vi "Fit_and_Size.vi"(0 "G2":dbl[](array[numeric]), 1 "A tau":dbl[](array[numeric]), 2 "Angle (degrees)":dbl=90.0, 5 "A(tau)":bool, 9 "bin mean":dbl, 11 "Time":dbl[](array[numeric])) -> (3 "Cumulant Fit":T1, 4 "Best Exponential Fit":dbl[](array[numeric]), 10 "Best Polynomial Fit":dbl[](array[numeric]), 12 "x < 0?":bool, 14 "ln(x)/2":dbl[](array[numeric]), 15 "Fit":T2)   [LabVIEW 2022 SP3]
uses:
  <vilib>/Analysis/6fits.llb/Curve Fitting Criteria.ctl
  <vilib>/Analysis/NI_AALPro.lvlib
panel:
  out "Waveform Graph":dbl[](graph)
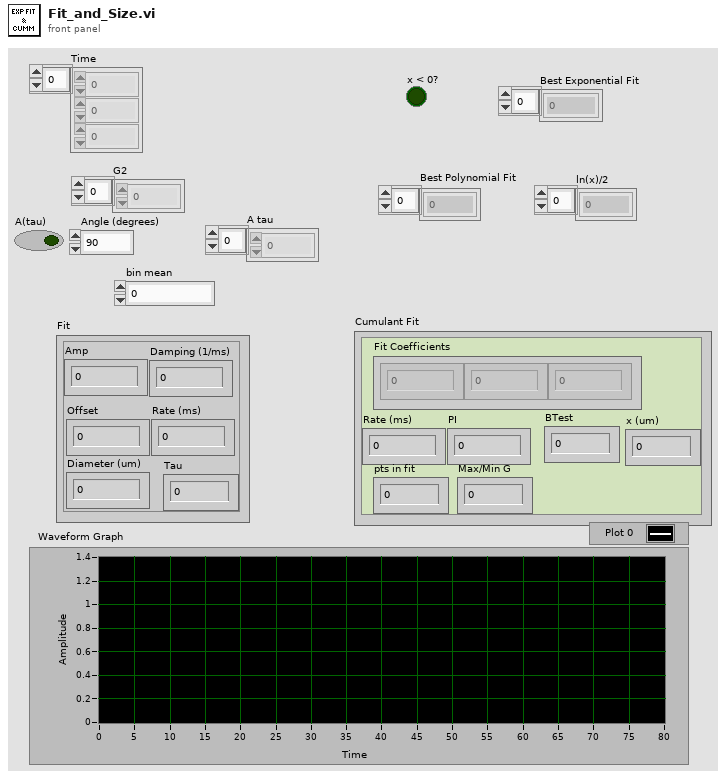
[diagram p1: front panel]
types:
  T1 = cluster{"Fit Coefficients":dbl[], "Rate (ms)":dbl, "PI":dbl, "BTest":dbl, "x (um)":dbl, "pts in fit":dbl, "Max/Min G":dbl}
  T2 = cluster{"Amp":dbl, "Offset":dbl, "Damping (1/ms)":dbl, "Rate (ms)":dbl, "Diameter (um)":dbl, "Tau":dbl}
  T3 = cluster{"Boltzmans ":dbl, "Temp K":dbl, "Viscosity":dbl, "lamda (m)":dbl, "n":dbl}
  T4 = cluster{"amp min":dbl, "amp max":dbl, "damping min":dbl, "damping max":dbl, "offset min":dbl, "offset max":dbl}
  T5 = typedef "NI_AALPro.lvlib/Curve Fitting Criteria.ctl" = u16
  T6 = cluster{"Polynomial Coefficients":dbl[], "rate":dbl, "PI":dbl, "Bratio":dbl, "x":dbl, i32, dbl}
  T7 = cluster{"amplitude":dbl, "offset":dbl, "damping":dbl, dbl, "size (um) ":dbl, "damping":dbl}
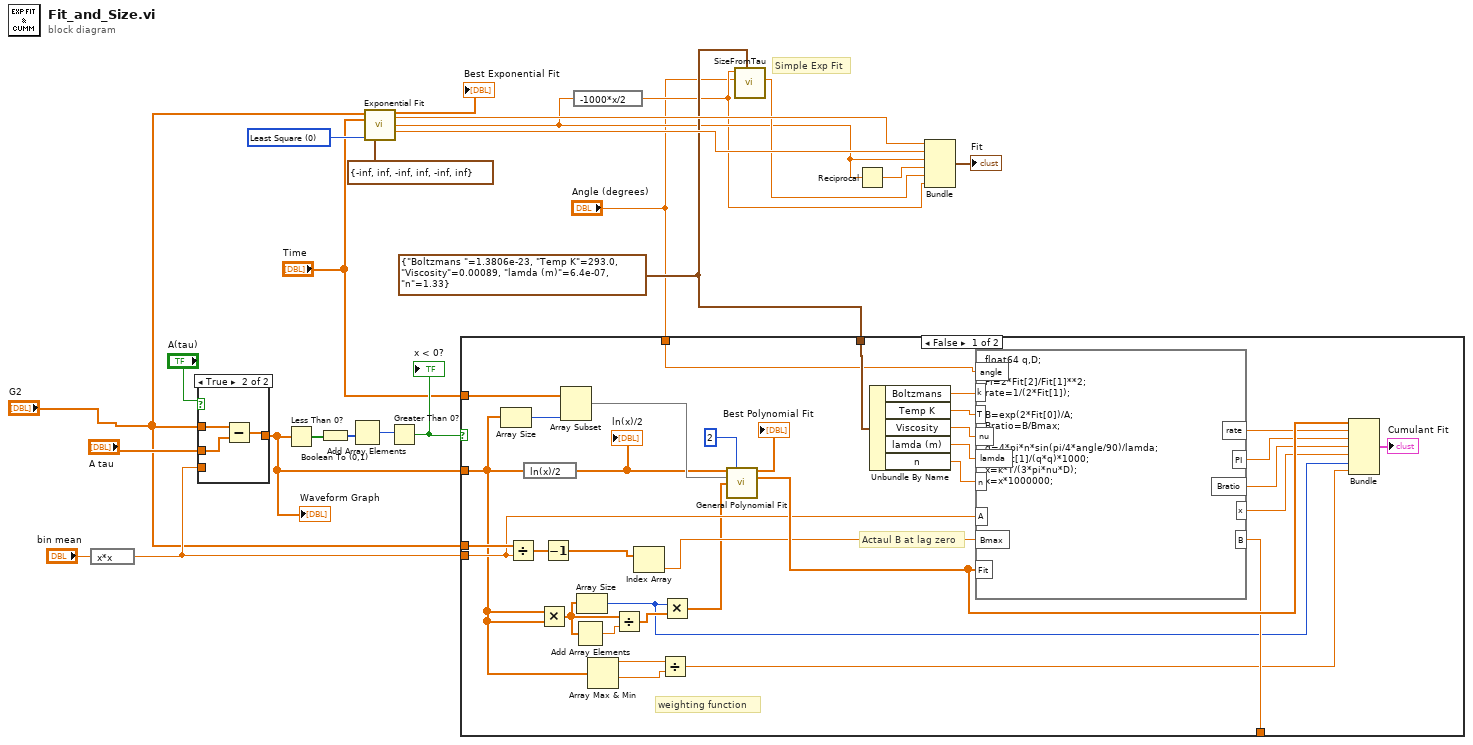
[diagram p0: block diagram]
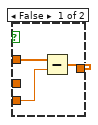
[diagram p2: hidden frame]
diagram:
  w12 = T3 {"Boltzmans "=1.3806e-23, "Temp K"=293.0, "Viscosity"=0.00089, "lamda (m)"=6.4e-07, "n"=1.33}
  w23 = T5 0 items=["Least Square", "Least Absolute Residual", "Bisquare"] ("method")
  # "Simple Exp Fit"
  n1 = expression code="x*x"("bin mean") -> (w3:dbl)
  n2 = case shown="True" "A(tau)" {
    tunnel: w3 -> [w26 _]
    tunnel: "G2" -> [w25 w28]
    tunnel: [w24 w29] -> w6
    tunnel: "A tau" -> [_ w27]
    frame False {
      n3 = Subtract(x=w25, y=w26) -> (x-y=w24:dbl[])
    }
    frame True {
      n4 = Subtract(x=w28, y=w27) -> (x-y=w29:dbl[])
    }
  }
  "Waveform Graph" <- w6
  n5 = Less Than 0?(x=w6) -> (x < 0?=w18:bool[])
  n6 = Boolean To (0,1)(Boolean=w18) -> (0, 1=w17:i16[])
  n7 = Add Array Elements(numeric array=w17) -> (sum=w16:i16)
  n8 = call <vilib>:"Exponential Fit.vi"("Y"="G2", "X"="Time", "method"=w23, "parameter bounds"=T4 {"amp min"=-inf, "amp max"=inf, "damping min"=-inf, "damping max"=inf, "offset min"=-inf, "offset max"=inf}) -> ("Best Exponential Fit"=→"Best Exponential Fit":dbl[], "amplitude"=w21:dbl, "damping"=w10:dbl, "offset"=w20:dbl)  [unwired: 6 in, 2 out]
  n9 = Greater Than 0?(x=w16) -> (x > 0?=w15:bool)
  "x < 0?" <- w15
  n10 = case shown="False" w15 {
    tunnel: w6 -> [w34 _]
    tunnel: "Time" -> [w36 _]
    tunnel: [w56 _] -> _
    tunnel: "G2" -> [w54 _]
    tunnel: w3 -> [w37 _]
    tunnel: w12 -> [w49 _]
    tunnel: "Angle (degrees)" -> [w30 _]
    frame False {
      # "Actaul B at lag zero"
      # "weighting function"
      n11 = Array Size(array=w34) -> (size(s)=w33:i32)
      n12 = Divide(x=w54, y=w37) -> (x/y=w53:dbl[])
      n13 = expression code="ln(x)/2"(w34) -> (w32:dbl[])
      "ln(x)/2" <- w32
      n14 = Multiply(x=w34, y=w34) -> (x*y=w51:dbl[])
      n15 = Decrement(x=w53) -> (x-1=w39:dbl[])
      n16 = Array Subset(array=w36, length=w33) -> (w35:dbl[])  [unwired: 1 in]
      n17 = Add Array Elements(numeric array=w51) -> (sum=w55:dbl)
      n18 = Array Size(array=w51) -> (size(s)=w43:i32)
      n19 = Array Max & Min(array=w34) -> (max value=w42:dbl, min value=w41:dbl)  [unwired: 2 out]
      n20 = Divide(x=w51, y=w55) -> (x/y=w50:dbl[])
      n21 = Index Array(array=w39) -> (element=w38:dbl)  [unwired: 1 in]
      n22 = Divide(x=w42, y=w41) -> (x/y=w40:dbl)
      n23 = Multiply(x=w43, y=w50) -> (x*y=w31:dbl[])
      n24 = call <vilib>:"General Polynomial Fit.vi"("Y"=w32, "polynomial order"=2, "X"=w35, "Weight"=w31) -> ("Best Polynomial Fit"=→"Best Polynomial Fit":dbl[], "Polynomial Coefficients"=w61:dbl[])  [unwired: 8 in, 2 out]
      n25 = Unbundle By Name(w49) -> ("Boltzmans"=w48:dbl, "Temp K"=w47:dbl, "Viscosity"=w46:dbl, "lamda (m)"=w45:dbl, "n"=w44:dbl)
      n26 = formula code="float64 q,D;\n\nPI=2*Fit[2]/Fit[1]**2;\nrate=1/(2*Fit[1]);\n\nB=exp(2*Fit[0])/A;\nBratio=B/Bmax;\n\nq=4*pi*n*sin(pi/4*angle/90)/lamda;\nD=-Fit[1]/(q*q)*1000;\nx=k*T/(3*pi*nu*D);\nx=x*1000000;"("Fit"=w61, "A"=w37, "Bmax"=w38, "T"=w47, "nu"=w46, "k"=w48, "lamda"=w45, "n"=w44, "angle"=w30) -> ("PI"=w59:dbl, "rate"=w60:dbl, "Bratio"=w58:dbl, "B"=w56:dbl, "x"=w52:dbl)
      n27 = Bundle("Polynomial Coefficients"=w61, "rate"=w60, "PI"=w59, "Bratio"=w58, "x"=w52, w43, w40) -> (→"Cumulant Fit":T6)  [unwired: 1 in]
    }
    frame True {
    }
  }
  n28 = expression code="-1000*x/2"(w10) -> (w9:dbl)
  n29 = call "SizeFromTau.vi"("Variables"=w12, "Angle (degrees)"="Angle (degrees)", "tau 1/s"=w9) -> ("size (um)"=w11:dbl)  [unwired: 7 in, 1 out]
  n30 = Reciprocal(x=w10) -> (1/x=w19:dbl)
  n31 = Bundle("amplitude"=w21, "offset"=w20, "damping"=w10, w19, "size (um)"=w11, "damping"=w9) -> (→"Fit":T7)  [unwired: 1 in]
